vi "Re_run_Gnuplot.vi"(0 "Plot folder (dialog if empty)":path) -> ()   [LabVIEW 2010]
panel:
  in  "Data file":string
  in  "stop":bool
  in  "OK Button":bool
  in  "Gnuplot script file":string
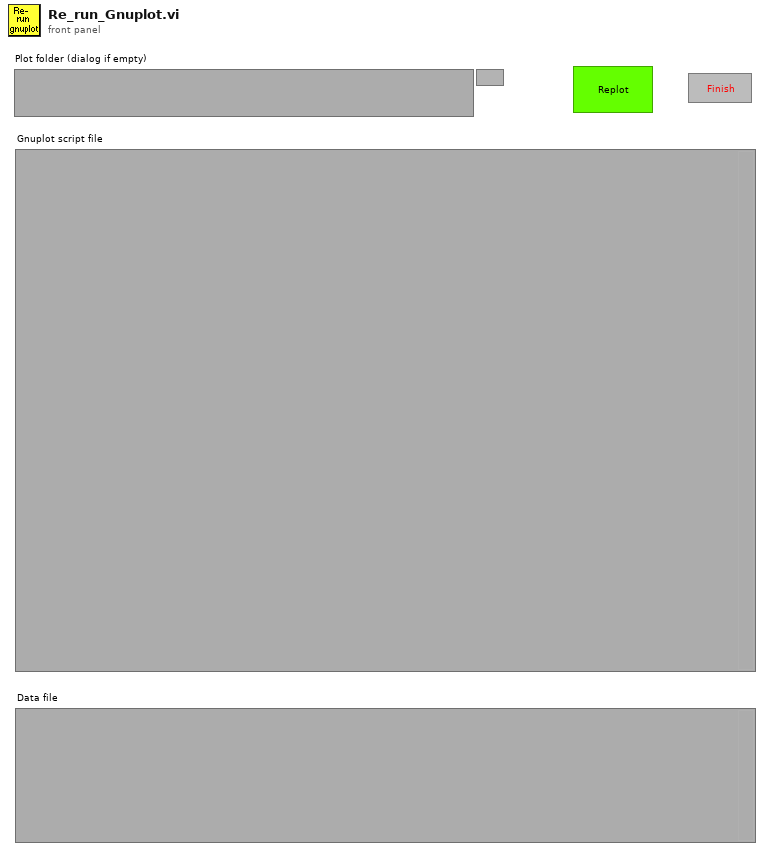
[diagram p1: front panel]
types:
  T1 = enum32{"existing file", "new file", "new or existing file", "existing dir", "new dir", "new or existing dir", "existing file (use LLBs)", "new file (use LLBs)", "new or existing file (use LLBs)", "new or existing file or directory (use LLBs)"}
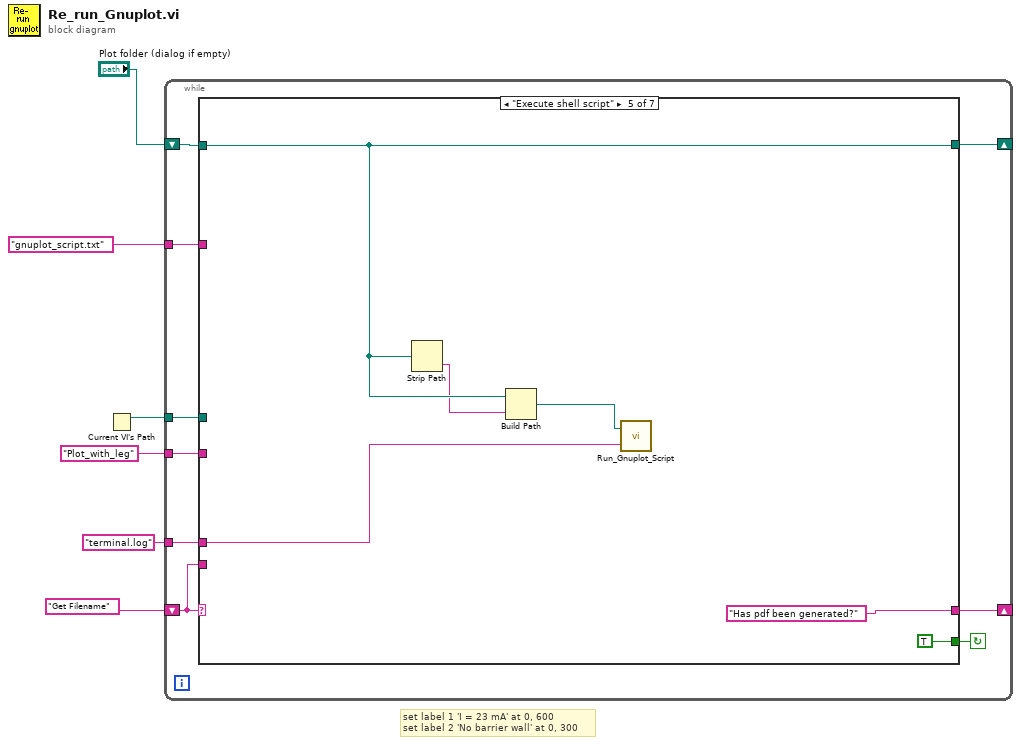
[diagram p0: block diagram]
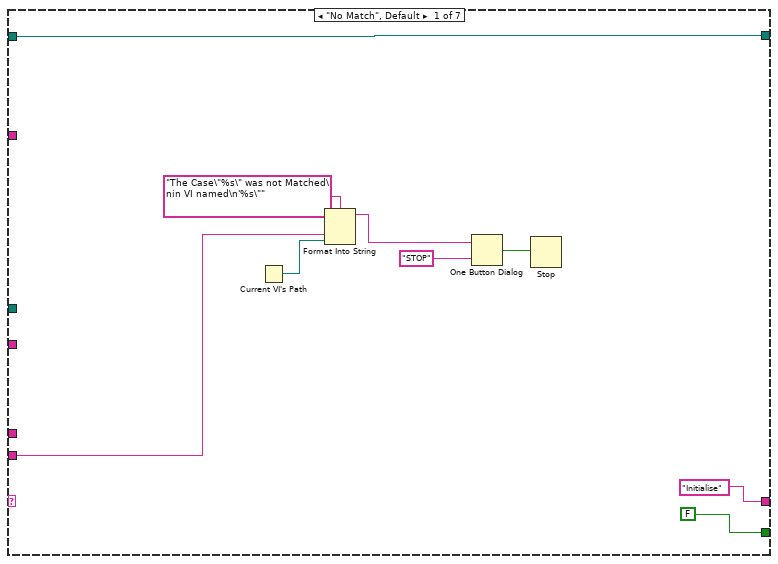
[diagram p2: hidden frame]
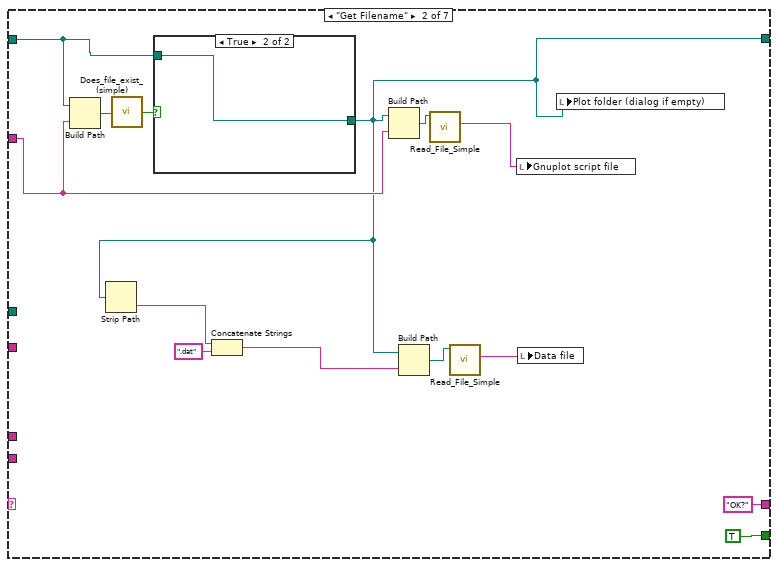
[diagram p3: hidden frame]
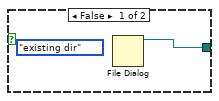
[diagram p4: hidden frame]
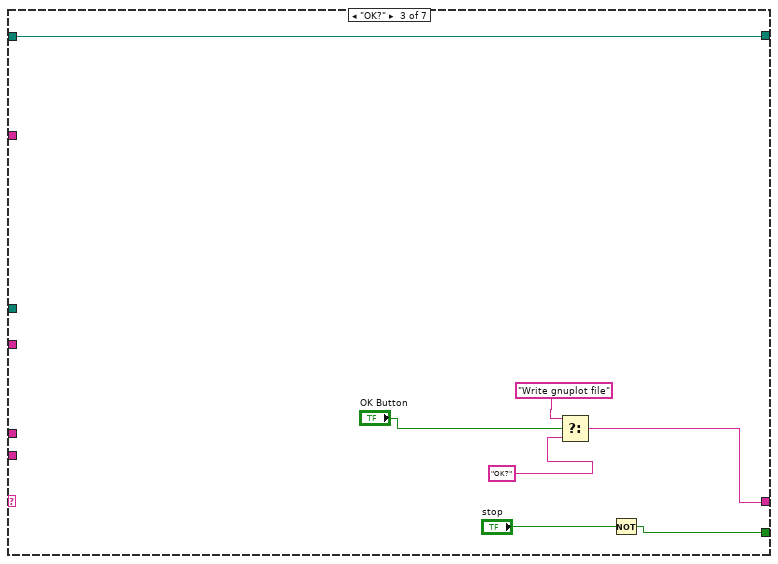
[diagram p5: hidden frame]
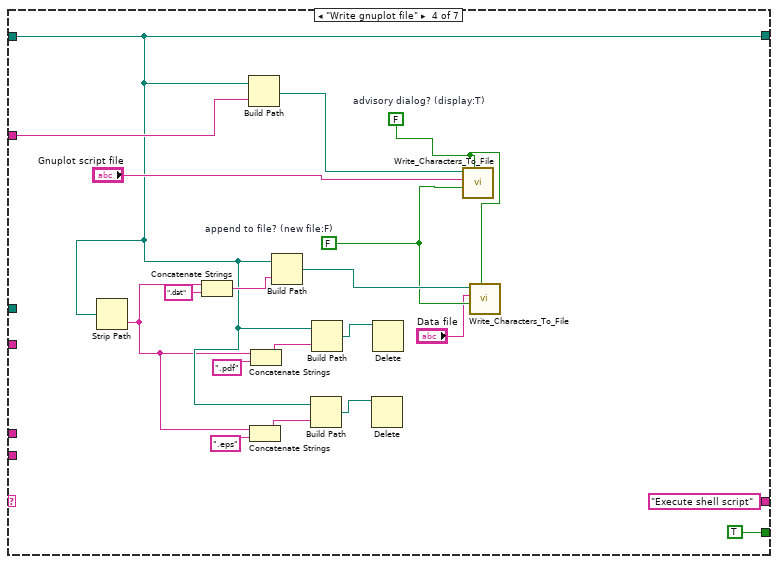
[diagram p6: hidden frame]
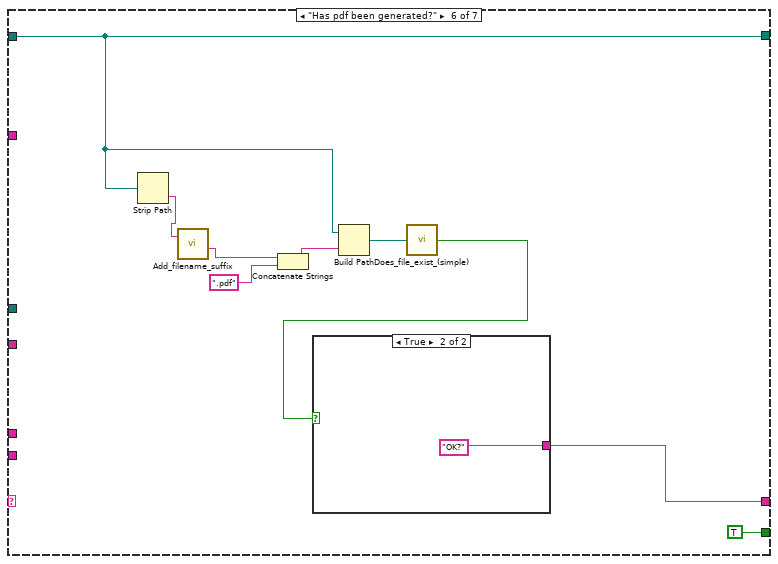
[diagram p7: hidden frame]
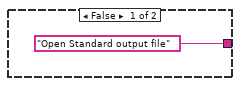
[diagram p8: hidden frame]
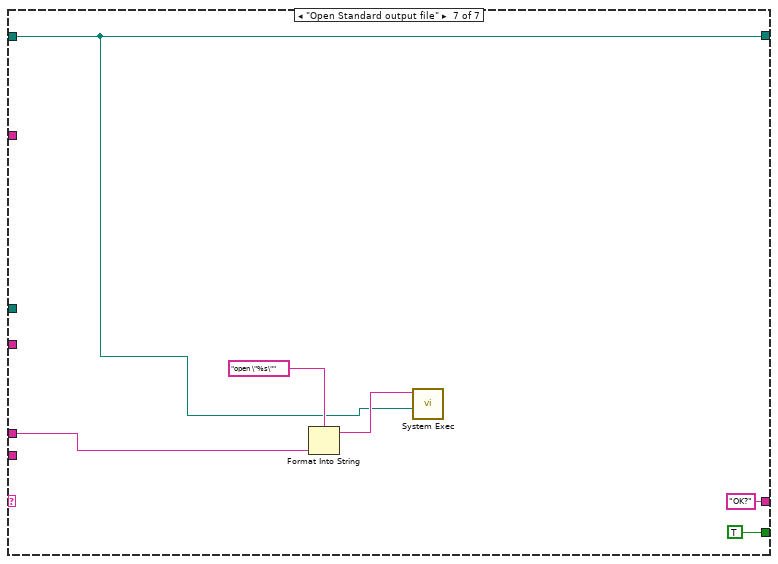
[diagram p9: hidden frame]
diagram:
  # "set label 1 'I = 23 mA' at 0, 600\nset label 2 'No barrier wall' at 0, 300"
  n1 = Current VI's Path() -> (path=w5:path)
  n2 = while {
    shift-left: "Get Filename" -> [w13]
    shift-right: [w14] -> _
    tunnel: w5 -> [w12]
    shift-right: [w11] -> _
    shift-left: "Plot folder (dialog if empty)" -> [w10]
    tunnel: "Plot_with_leg" ("name or relative path") -> [w9]
    tunnel: "terminal.log" -> [w8]
    tunnel: "gnuplot_script.txt" -> [w7]
    stop <- w15 continue-if-true
    n3 = case shown="\"Execute shell script\"" w13 {
      tunnel: [FALSE TRUE ("Top Level") w41 TRUE ("Top Level") TRUE ("Top Level") TRUE ("Top Level") TRUE ("Top Level")] -> w15
      tunnel: ["Initialise" "OK?" ("t") w47 "Execute shell script" ("t") "Has pdf been generated?" ("t") w78 "OK?" ("t")] -> w14
      tunnel: w13 -> [w19 _ _ _ _ _ _]
      tunnel: w12 -> [_ _ _ _ _ _ _]
      tunnel: [w16 w30 w44 w49 w69 w73 w84] -> w11
      tunnel: w10 -> [w16 w34 w44 w49 w69 w73 w84]
      tunnel: w9 -> [_ _ _ _ _ _ _]
      tunnel: w8 -> [_ _ _ _ w70 _ w86]
      tunnel: w7 -> [_ w33 _ w62 _ _ _]
      frame "No Match", Default {
        n4 = Current VI's Path() -> (path=w18:path)
        n5 = Format Into String(format string="The Case\"%s\" was not Matched\nin VI named\n'%s\"" ("Format String"), w19, w18) -> (resulting string=w22:string)  [unwired: 2 in, 1 out]
        n6 = One Button Dialog(message=w22, button name ("OK")="STOP") -> (true=w20:bool)
        n7 = Stop(stop? (T)=w20) -> ()
      }
      frame "Get Filename" {
        n8 = Build Path(base path=w34, name or relative path=w33) -> (appended path=w32:path)
        n9 = call "Does_file_exist_(simple).vi"("Pathname"=w32) -> ("exists?"=w31:bool)
        n10 = case shown="True" w31 {
          tunnel: [w39 w40] -> w30
          tunnel: w34 -> [_ w40]
          frame False {
            (unwired) T1."existing dir" ("select mode (2)")
            n11 = File Dialog() -> (3:w39:path)  [unwired: 1 in, 9 out]
          }
          frame True {
          }
        }
        n12 = Strip Path(path=w30) -> (name=w29:string)  [unwired: 1 out]
        n13 = Concatenate Strings(w29, ".dat" ("string")) -> (w27:string)
        n14 = Build Path(base path=w30, name or relative path=w33) -> (appended path=w35:path)
        n15 = Build Path(base path=w30, name or relative path=w27) -> (appended path=w26:path)
        n16 = call "Read_File_Simple.vi"("Filename"=w35) -> ("string"=w37:string)  [unwired: 2 in, 7 out]
        n17 = call "Read_File_Simple.vi"("Filename"=w26) -> ("string"=w25:string)  [unwired: 2 in, 7 out]
        n18 = local write "Gnuplot script file"(w37) -> ()
        n19 = local write "Data file"(w25) -> ()
        n20 = local write "Plot folder (dialog if empty)"(w30) -> ()
      }
      frame "OK?" {
        n21 = Select(t="Write gnuplot file", s="OK Button", f="OK?") -> (s? t:f=w47:string)
        n22 = Not(x="stop") -> (.not. x?=w41:bool)
      }
      frame "Write gnuplot file" {
        w58 = FALSE  # append to file? (new file:F)
        w57 = FALSE  # advisory dialog? (display:T)
        n23 = Strip Path(path=w49) -> (name=w48:string)  [unwired: 1 out]
        n24 = Concatenate Strings(w48, ".dat" ("string")) -> (w60:string)
        n25 = Build Path(base path=w49, name or relative path=w62) -> (appended path=w66:path)
        n26 = Concatenate Strings(w48, ".eps" ("string")) -> (w50:string)
        n27 = Concatenate Strings(w48, ".pdf" ("string")) -> (w55:string)
        n28 = Build Path(base path=w49, name or relative path=w60) -> (appended path=w59:path)
        n29 = Build Path(base path=w49, name or relative path=w50) -> (appended path=w52:path)
        n30 = Build Path(base path=w49, name or relative path=w55) -> (appended path=w53:path)
        n31 = Delete(path (use dialog)=w52) -> ()  [unwired: 1 in, 6 out]
        n32 = Delete(path (use dialog)=w53) -> ()  [unwired: 1 in, 6 out]
        n33 = call "Write_Characters_To_File.vi"("file path (dialog if empty)"=w66, "advisory dialog? (display:T)"=w57, "character string"="Gnuplot script file", "append to file? (new file:F)"=w58) -> ()  [unwired: 1 in, 4 out]
        n34 = call "Write_Characters_To_File.vi"("file path (dialog if empty)"=w59, "advisory dialog? (display:T)"=w57, "character string"="Data file", "append to file? (new file:F)"=w58) -> ()  [unwired: 1 in, 4 out]
      }
      frame "Execute shell script" {
        n35 = Strip Path(path=w69) -> (name=w68:string)  [unwired: 1 out]
        n36 = Build Path(base path=w69, name or relative path=w68) -> (appended path=w67:path)
        n37 = call "Run_Gnuplot_Script.vi"("logfileName"=w70, "workingDirectory"=w67) -> ()
      }
      frame "Has pdf been generated?" {
        n38 = Strip Path(path=w73) -> (name=w75:string)  [unwired: 1 out]
        n39 = call "Add_filename_suffix.vi"("Filename"=w75) -> ("Base name"=w74:string)  [unwired: 1 in, 3 out]
        n40 = Concatenate Strings(w74, ".pdf" ("string")) -> (w81:string)
        n41 = Build Path(base path=w73, name or relative path=w81) -> (appended path=w79:path)
        n42 = call "Does_file_exist_(simple).vi"("Pathname"=w79) -> ("exists?"=w77:bool)
        n43 = case shown="True" w77 {
          tunnel: ["Open Standard output file" ("f") "OK?" ("t")] -> w78
          frame False {
          }
          frame True {
          }
        }
      }
      frame "Open Standard output file" {
        n44 = Format Into String(format string="open \"%s\"", w86) -> (resulting string=w85:string)  [unwired: 2 in, 1 out]
        n45 = call <vilib>:"System Exec.vi"("working directory"=w84, "command line"=w85) -> ()  [unwired: 4 in, 6 out]
      }
    }
  }
